vi "Host - Primary BMS Data (SubVI).vi"(11 "Sring Data":string) -> (1 "SOC":dbl, 2 "Current":dbl, 3 "Voltage":dbl, 4 "Temperature":dbl)   [LabVIEW 2021]
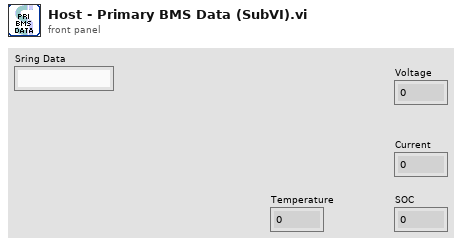
[diagram p1: front panel]
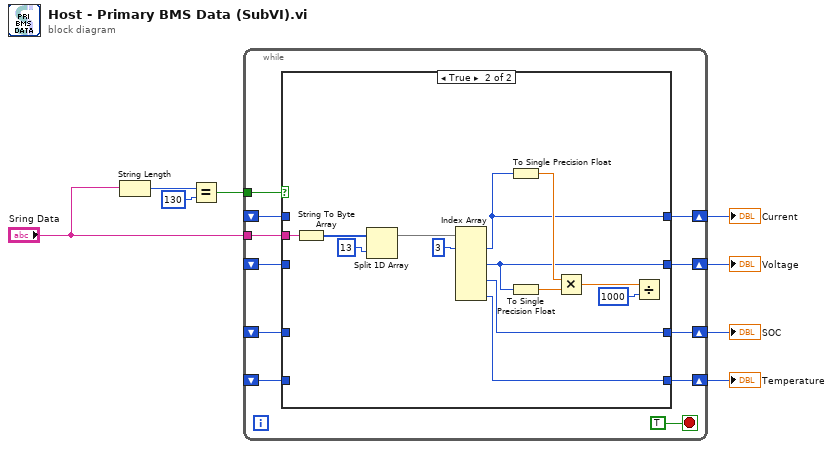
[diagram p0: block diagram]
diagram:
  n1 = String Length(string="Sring Data") -> (length=w8:i32)
  n2 = Equal?(x=w8, y=130) -> (x = y?=w1:bool)
  n3 = while {
    tunnel: "Sring Data" -> [w19]
    shift-right: [w17] -> w4
    shift-left: _ -> [w13]
    shift-right: [w18] -> w5
    shift-left: _ -> [w12]
    shift-right: [w15] -> w2
    shift-left: _ -> [w11]
    shift-right: [w16] -> w3
    shift-left: _ -> [w10]
    tunnel: w1 -> [w14]
    stop <- TRUE stop-if-true
    n4 = case shown="True" w14 {
      tunnel: w19 -> [_ w29]
      tunnel: [w22 w27] -> w18
      tunnel: [w23 w26] -> w17
      tunnel: [w20 w25] -> w16
      tunnel: [w21 w24] -> w15
      tunnel: w13 -> [w23 _]
      tunnel: w12 -> [w22 _]
      tunnel: w11 -> [w21 _]
      tunnel: w10 -> [w20 _]
      frame False {
      }
      frame True {
        n5 = String To Byte Array(string=w29) -> (unsigned byte array=w30:u8[])
        n6 = Split 1D Array(array=w30, index=13) -> (first subarray=w35:u8[])  [unwired: 1 out]
        n7 = Index Array(array=w35, index #1=3 ("index")) -> (element #1=w26:u8, element #3=w27:u8, element #5=w24:u8, element #7=w25:u8)  [unwired: 6 in, 3 out]
        n8 = To Single Precision Float(number=w26) -> (single precision float=w33:sgl)
        n9 = To Single Precision Float(number=w27) -> (single precision float=w32:sgl)
        n10 = Multiply(x=w33, y=w32) -> (x*y=w31:sgl)
        n11 = Divide(x=w31, y=u16 1000) -> ()  [unwired: 1 out]
      }
    }
  }
  "Voltage" <- w5
  "Current" <- w4
  "SOC" <- w2
  "Temperature" <- w3
